vi "GetInstVisaHandle.vi"(8 "error in (no error)":errorcluster, 11 "NetA_AgNA in":refnum<class "NetA_AgNA.lvclass">) -> (0 "error out":errorcluster, 2 "instrument handle":refnum<k15>, 3 "NetA_AgNA out":refnum<class "NetA_AgNA.lvclass">)   [LabVIEW 2014, in "NetA_AgNA.lvclass"]
uses:
  NetA_AgNA.lvclass
  NetA_AgNA.lvclass/NetA_AgNA.ctl
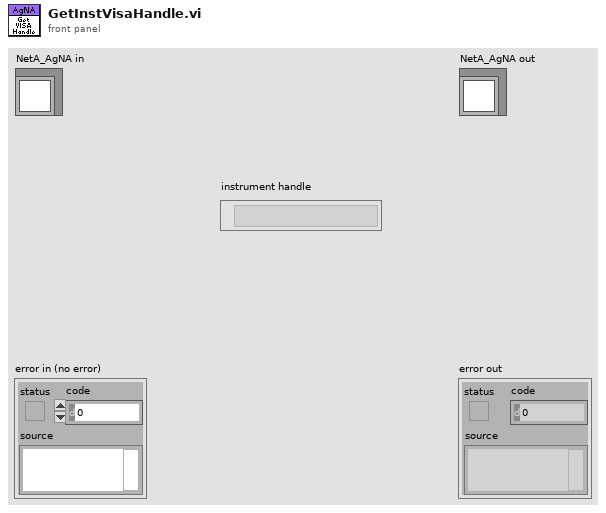
[diagram p1: front panel]
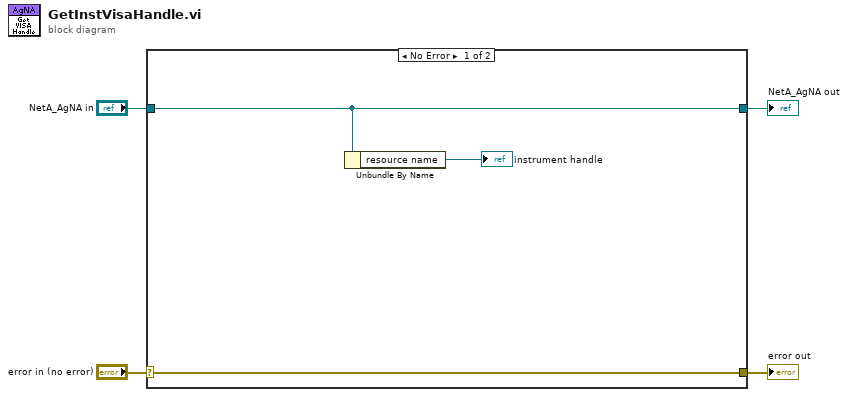
[diagram p0: block diagram]
diagram:
  n1 = case shown="No Error" "error in (no error)" {
    selector: "error in (no error)" -> [w7 w9]
    tunnel: [w7 w9] -> w3
    tunnel: [w6 w8] -> w1
    tunnel: "NetA_AgNA in" -> [w6 w8]
    frame No Error {
      n2 = Unbundle By Name(w6) -> ("resource name"=→"instrument handle":refnum<k15>)
    }
    frame Error {
    }
  }
  "error out" <- w3
  "NetA_AgNA out" <- w1
